vi "Get Service Descriptor.vi"(8 "error in":errorcluster) -> (0 "error out":errorcluster, 3 "service descriptor":T1)   [LabVIEW 2022 SP3, in "Efficiency_Class D Amplifier.lvlib"]
uses:
  Efficiency_Class D Amplifier.lvlib
  <vilib>/Plug-In SDKs/Measurements/NI Measurement Plug-In SDK.lvlib
  <vilib>/Plug-In SDKs/Measurements/Helpers/TypeDefs/Measurement Details.ctl
  <vilib>/Plug-In SDKs/Measurements/Helpers/TypeDefs/Measurement Annotation.ctl
  <vilib>/Plug-In SDKs/Measurements/Helpers/TypeDefs/Service Descriptor.ctl
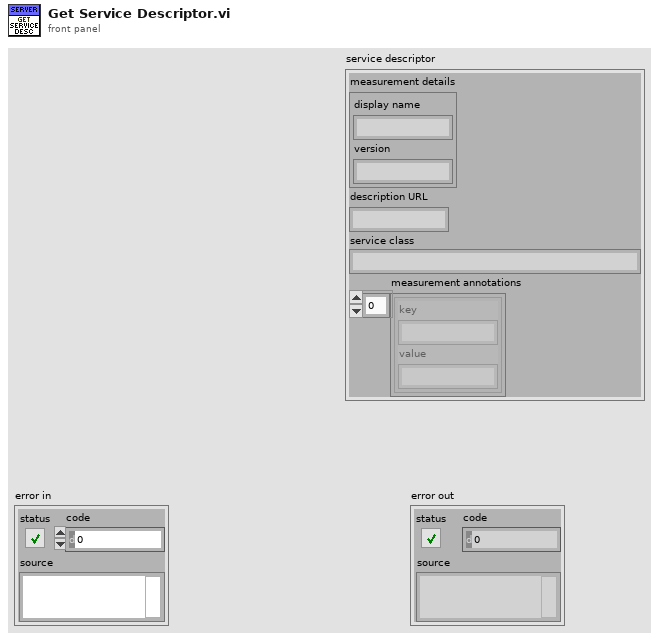
[diagram p1: front panel]
types:
  T1 = typedef "NI Measurement Plug-In SDK.lvlib/Service Descriptor.ctl" = cluster{"measurement details":T2, "description URL":string, "service class":string, "measurement annotations":T3[]}
  T2 = typedef "NI Measurement Plug-In SDK.lvlib/Measurement Details.ctl" = cluster{"display name":string, "version":string}
  T3 = typedef "NI Measurement Plug-In SDK.lvlib/Measurement Annotation.ctl" = cluster{"key":string, "value":string}
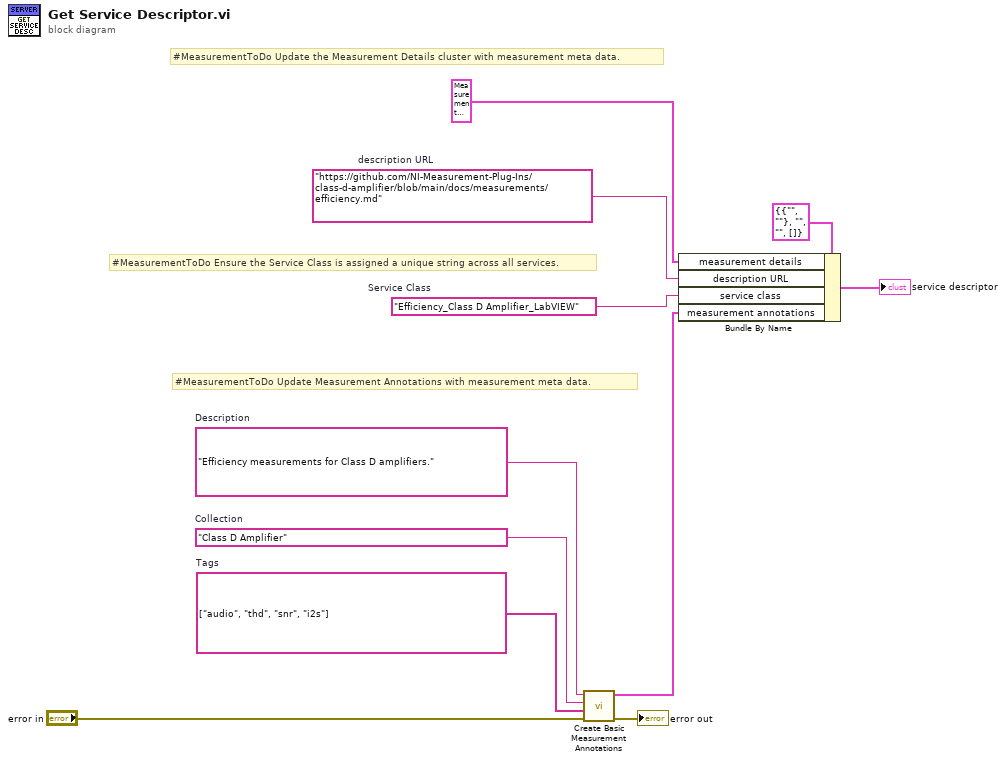
[diagram p0: block diagram]
diagram:
  w1 = "https://github.com/NI-Measurement-Plug-Ins/class-d-amplifier/blob/main/docs/measurements/efficiency.md"  # description URL
  w7 = string[] ["audio", "thd", "snr", "i2s"]  # Tags
  w8 = "Class D Amplifier"  # Collection
  w9 = "Efficiency measurements for Class D amplifiers."  # Description
  w3 = "Efficiency_Class D Amplifier_LabVIEW"  # Service Class
  # "#MeasurementToDo Update Measurement Annotations with measurement meta data."
  # "#MeasurementToDo Ensure the Service Class is assigned a unique string across all services."
  # "#MeasurementToDo Update the Measurement Details cluster with measurement meta data."
  n1 = call <vilib>:"Create Basic Measurement Annotations.vi"("error in"="error in", "tags"=w7, "collection"=w8, "description"=w9) -> ("error out"=→"error out":errorcluster, "measurement annotations"=w2:T3[])  [unwired: 6 in]
  n2 = Bundle By Name(cluster=T1 {"measurement details"={"display name"="", "version"=""}, "description URL"="", "service class"="", "measurement annotations"=[]} ("service descriptor"), "measurement details"=T2 {"display name"="Efficiency", "version"="1.0.0"} ("Measurement Details"), "description URL"=w1, "service class"=w3, "measurement annotations"=w2) -> (→"service descriptor":T1)
